vi "FA_AgentConfig_GetCloudKeys.vi"(8 "Error In":errorcluster) -> (0 "Error Out":errorcluster, 1 "Keys Empty?":bool, 2 "x-ni-api-key":string, 3 "x-ni-client-id":string, 5 "DeviceName":string)   [LabVIEW 2014, in "FA_AgentConfig.lvlib"]
doc: "Obtains the Cloud API keys from the agent configuration file. Also checks if either of the keys are empty."
uses:
  FA_AgentConfig.lvlib
  FA_LocalStore API/source/VI Source/FA_LSSpecialTypes.ctl
  FA_LocalStore API/source/VI Source/FA_LocalStore.lvlib
  FA_NativeTypes API/source/VI Source/FA_NativeTypes.lvlib
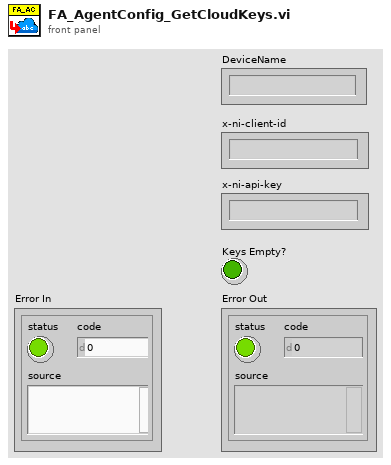
[diagram p1: front panel]
types:
  T1 = typedef "FA_LocalStore.lvlib/FA_LSSpecialTypes.ctl" = string
  T2 = typedef "FA_NativeTypes.lvlib/FA_Config.ctl" = cluster{"Id":string, "Name":T1, "Parameter":cluster{"Name":string, "Value":string}[], "Account":string, "CreateDate":string, "LastModified":string}
  T3 = typedef "FA_AgentConfig.lvlib/FA_AgentConfig.ctl" = cluster{"x-ni-client-id":string, "x-ni-apikey":string, "CloudLookupTime":u32, "Debug":bool, "DeviceName":string}
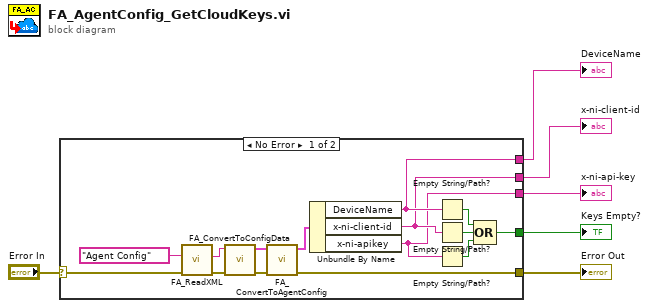
[diagram p0: block diagram]
diagram:
  n1 = case shown="No Error" "Error In" {
    selector: "Error In" -> [w20 w22]
    tunnel: [w16 w22] -> w5
    tunnel: [w8 _] -> w4
    tunnel: [w7 _] -> w3
    tunnel: [w10 _] -> w2
    tunnel: [w9 _] -> w1
    frame No Error {
      n2 = call "FA_ReadXML.vi"("Error In"=w20, "Special Type"=T1 "Agent Config") -> ("Error Out"=w19:errorcluster, "XML String"=w18:string)  [unwired: 6 in]
      n3 = call "FA_ConvertToConfigData.vi"("Error In"=w19, "XML String"=w18) -> ("Error Out"=w17:errorcluster, "ConfigData"=w15:T2)  [unwired: 8 in]
      n4 = call "FA_ConvertToAgentConfig.vi"("Error In"=w17, "Config"=w15) -> ("Error Out"=w16:errorcluster, "AgentConfig"=w14:T3)  [unwired: 8 in]
      n5 = Unbundle By Name(w14) -> ("DeviceName"=w9:string, "x-ni-client-id"=w8:string, "x-ni-apikey"=w7:string)
      n6 = Empty String/Path?(string/path=w9) -> (empty?=w13:bool)
      n7 = Empty String/Path?(string/path=w8) -> (empty?=w12:bool)
      n8 = Empty String/Path?(string/path=w7) -> (empty?=w11:bool)
      n9 = Compound Arithmetic op=OR(w13, w12, w11) -> (w10:bool)
    }
    frame Error {
    }
  }
  "Error Out" <- w5
  "x-ni-client-id" <- w4
  "x-ni-api-key" <- w3
  "Keys Empty?" <- w2
  "DeviceName" <- w1
